vi "LoadTerminalVI.vi"(4 "VI Reference":string, 5 "XRef":refnum<vi>) -> (0 "Clone Number":i16, 1 "error out":errorcluster, 2 "vi reference":refnum<vi>)   [LabVIEW 2012]
uses:
  CThread.lvlib
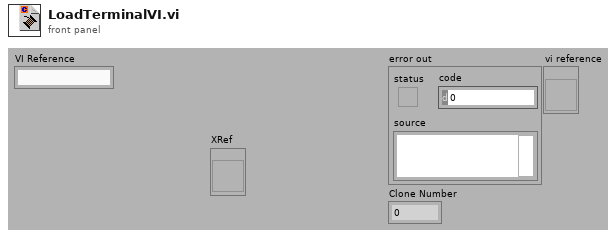
[diagram p1: front panel]
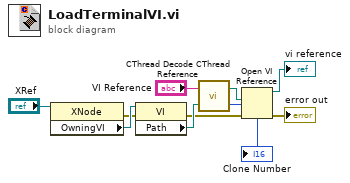
[diagram p0: block diagram]
diagram:
  n1 = property class="XNode"(reference="XRef") -> (error out=w8:errorcluster, "OwningVI"=w9:refnum<vi>)  [unwired: 1 in, 1 out]
  n2 = property class="VI"(reference=w9, error in=w8) -> (error out=w5:errorcluster, "Path"=w7:path)  [unwired: 1 out]
  n3 = call "CThread Decode CThread Reference.vi"("Owner Path"=w7, "CThread Reference"="VI Reference") -> ("Clone Number"=→"Clone Number":i16, "path"=w6:path)
  n4 = Open VI Reference(vi path=w6, error in (no error)=w5) -> (vi reference=→"vi reference":refnum<vi>, error out=→"error out":errorcluster)  [unwired: 4 in]
